vi "newUser.vi"() -> ()   [LabVIEW 2020, in "userLibrary.lvlib"]
uses:
  userLibrary.lvlib
  <vilib>/measure/mamon.llb/Trigger Detection for 1 Channel.vi
  <vilib>/addons/database/Connection.llb/DB Tools Open Connec (String).vi
  <vilib>/addons/database/_DB Variant To Data/Database Variant To Data.xnode
  <vilib>/addons/database/NI_Database_API.lvlib
  databaseLibrary.lvlib
  maintenanceLibrary.lvlib
  <vilib>/measure/NI_MAPro.lvlib
panel:
  out "status 2":bool
  out "status 1":bool
  out "Log Max row":i32
  in  "Cancel":bool
  in  "OK":bool
  in  "Is Admin?":enum32{"Yes", "No"}(radio)
  in  "Full Name":string
  in  "Confirm Password":string
  in  "Password":string
  in  "Username":string
  # "New User"
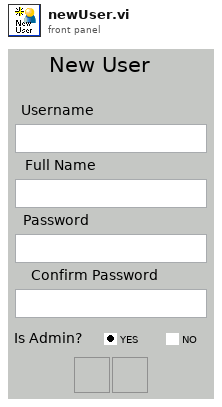
[diagram p1: front panel]
types:
  T1 = typedef "NI_Database_API.lvlib/Conn ObjectReference.ctl" = refnum<k1>
  T2 = cluster{"concatenated string":string, "date/time string":string, "date/time string":string, string}
  T3 = cluster{"Username":string, "Full Name":string, "Password":string, string}
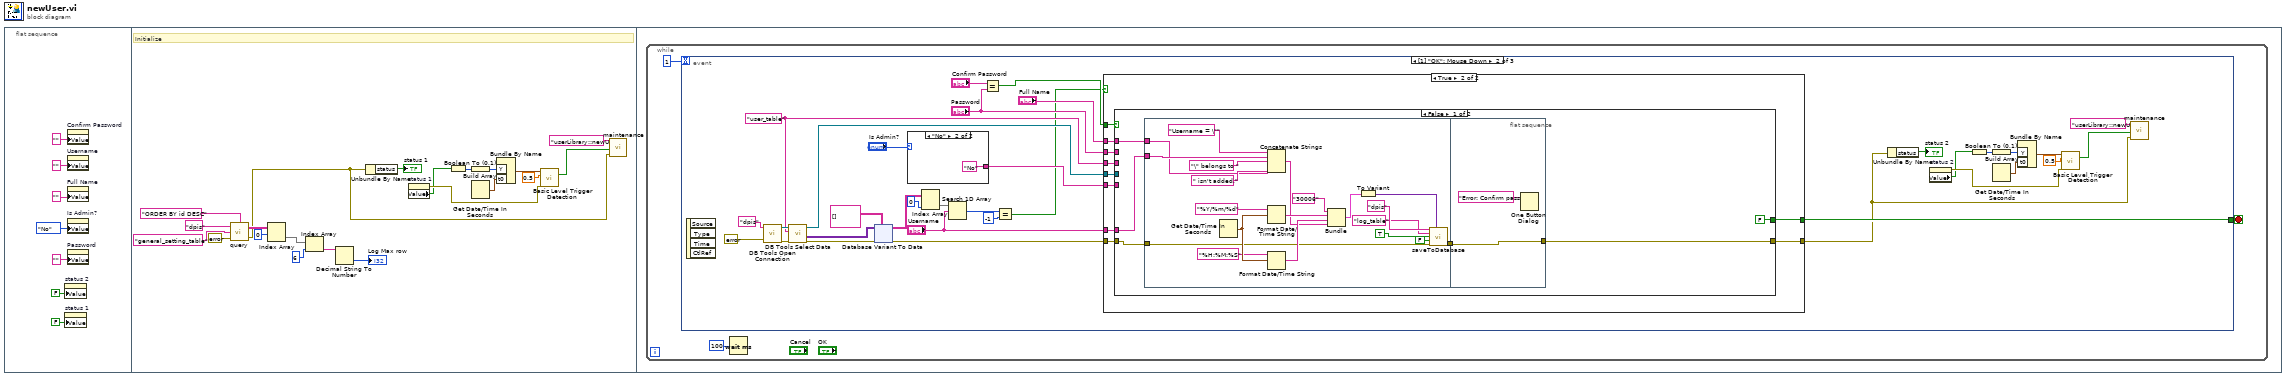
[diagram p0: block diagram]
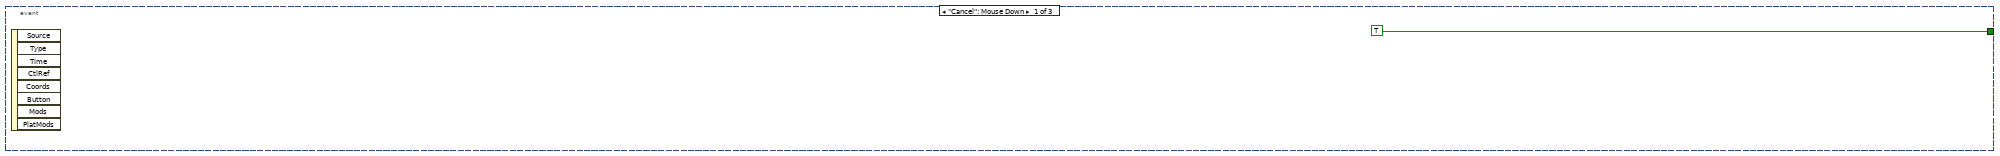
[diagram p2: hidden frame]
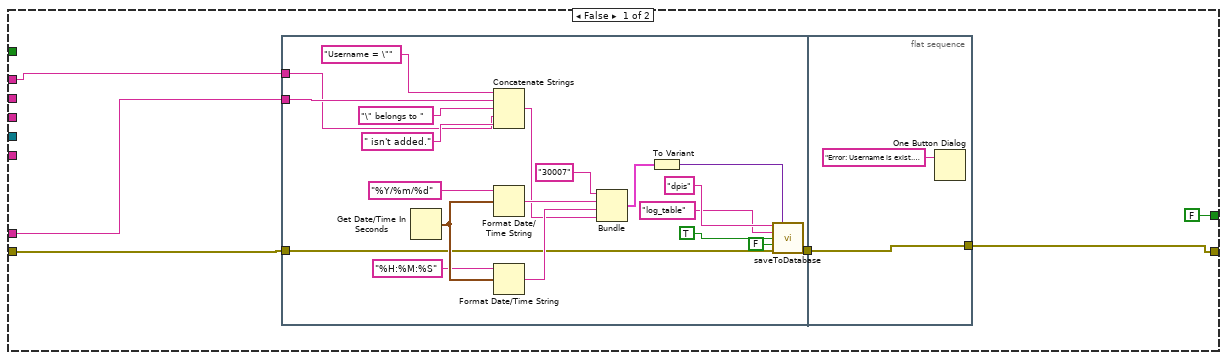
[diagram p3: hidden frame]
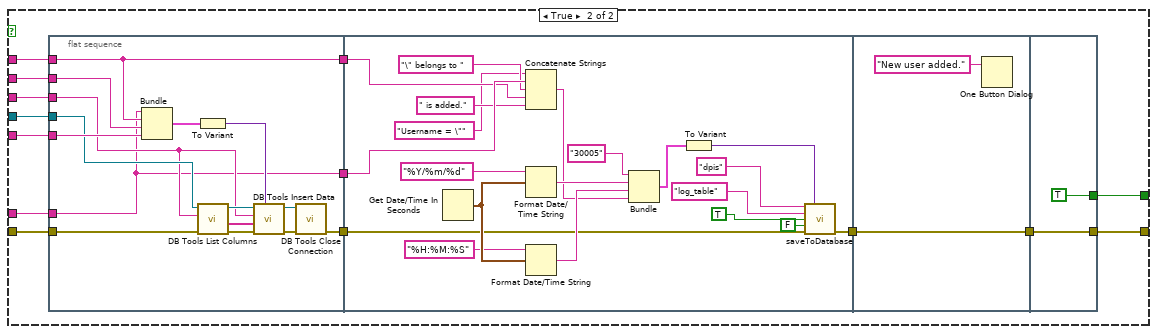
[diagram p4: hidden frame]
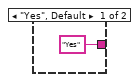
[diagram p5: hidden frame]
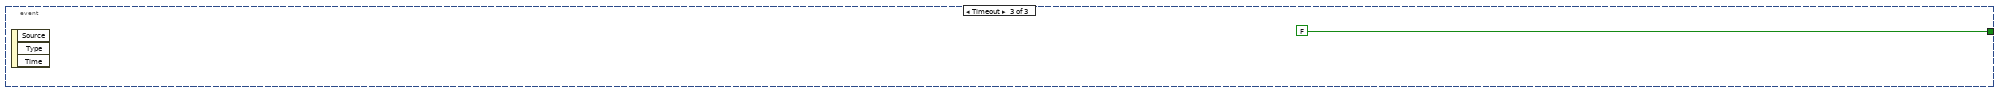
[diagram p6: hidden frame]
diagram:
  n1 = flat-sequence {
    frame #0 {
      n2 = property on="status 2" class="Bool (strict)"("Value"=FALSE ("status 2")) -> ()  [unwired: 2 in, 2 out]
      n3 = property on="status 1" class="Bool (strict)"("Value"=FALSE ("status 1")) -> ()  [unwired: 2 in, 2 out]
      n4 = property on="Confirm Password" class="Str"("Value"="" ("Username")) -> ()  [unwired: 2 in, 2 out]
      n5 = property on="Username" class="Str"("Value"="" ("Username")) -> ()  [unwired: 2 in, 2 out]
      n6 = property on="Full Name" class="Str"("Value"="" ("Full Name")) -> ()  [unwired: 2 in, 2 out]
      n7 = property on="Is Admin?" class="RadioBtnsControl (strict)"("Value"=enum32{"Yes", "No"}."No" ("Is Admin?")) -> ()  [unwired: 2 in, 2 out]
      n8 = property on="Password" class="Str"("Value"="" ("Username")) -> ()  [unwired: 2 in, 2 out]
    }
    frame #1 {
      # "Initialize"
      n9 = call "query.vi"("Condition"="ORDER BY id DESC", "errorIn"=errorcluster {"status"=FALSE, "code"=0, "source"=""} ("Error in"), "Table Name"="general_setting_table", "Connection Name"="dpis") -> ("errorOut"=w8:errorcluster, "data"=w28:string[][])
      n10 = Index Array(array=w28, index (row)=0) -> (element=w27:string[])  [unwired: 1 in]
      n11 = Index Array(array=w27, index=6) -> (element=w26:string)
      n12 = Decimal String To Number(string=w26) -> (number=→"Log Max row":i32)  [unwired: 2 in, 1 out]
      n13 = Unbundle By Name(w8) -> ("status"=→"status 1":bool)
      n14 = property on="status 1" class="Bool (strict)"() -> (error out=w16:errorcluster, "Value"=w15:bool)  [unwired: 2 in, 1 out]
      n15 = Boolean To (0,1)(Boolean=w15) -> (0, 1=w11:i16)
      n16 = Build Array(w11) -> (w13:i16[])
      n17 = Get Date/Time In Seconds() -> (seconds since 1Jan1904=w12:timestamp)
      n18 = Bundle By Name("Y"=w13, "t0"=w12) -> (w14:waveform(i16))  [unwired: 1 in]
      n19 = call-poly <vilib>:"Basic Level Trigger Detection.vi"("signal in"=w14, "level"=0.5, "error in (no error)"=w16) -> ("trigger detected?"=w17:bool)  [unwired: 10 in, 2 out]
      n20 = call "maintenance.vi"("errorIn"=w8, "status"=w17, "errorLocation"="userLibrary::newUser.vi::Initialize") -> ()  [unwired: 8 in, 1 out]
    }
    frame #2 {
      n21 = while {
        stop <- w30 stop-if-true
        n22 = event shown="[1] \"OK\": Mouse Down" {
          selector: _ -> [_ _ _]
          dyn-events: _ -> [_ _ _]
          timeout: 1 -> [_ _ _]
          tunnel: [TRUE w44 FALSE] -> w30
          event "Cancel": Mouse Down {
            n23 = event-data() -> ()  [unwired: 1 in, 8 out]
          }
          event "OK": Mouse Down {
            w57 = "user_table" ("Heat Table Name")
            n24 = event-data() -> ()  [unwired: 1 in, 4 out]
            n25 = call-poly <vilib>:"DB Tools Open Connection.vi"("error in (no error)"=errorcluster {"status"=FALSE, "code"=0, "source"=""}, "connection information"="dpis" ("Connection Name")) -> ("error out"=w61:errorcluster, "connection reference"=w60:T1)  [unwired: 6 in]
            n26 = call <vilib>:"DB Tools Select Data.vi"("error in (no error)"=w61, "table"=w57, "connection reference"=w60) -> ("error out"=w55:errorcluster, "data"=w56:variant[][], "connection reference out"=w58:T1)  [unwired: 3 in]
            n27 = xnode "Database Variant To Data"("database variant"=w56, "error in (no error)"=w55, "type"=string[][] []) -> ("data"=w52:string[][], "error out"=w54:errorcluster)
            n28 = case shown="\"No\"" "Is Admin?" {
              tunnel: ["Yes" "No"] -> w62
              frame "Yes", Default {
              }
              frame "No" {
              }
            }
            n29 = Index Array(array=w52, index (col)=0 ("disabled index (col)")) -> (element=w50:string[])  [unwired: 1 in]
            n30 = Search 1D Array(1D array=w50, element="Username") -> (index of element=w48:i32)  [unwired: 1 in]
            n31 = Equal?(x="Confirm Password", y="Password") -> (x = y?=w65:bool)
            n32 = Equal?(x=w48, y=-1) -> (x = y?=w46:bool)
            n33 = case shown="True" w46 {
              tunnel: w65 -> [_ w105]
              tunnel: "Full Name" -> [w69 w104]
              tunnel: "Password" -> [_ w103]
              tunnel: w62 -> [_ w102]
              tunnel: [FALSE w101] -> w44
              tunnel: w58 -> [_ w100]
              tunnel: [w70 w96] -> w33
              tunnel: w57 -> [_ w99]
              tunnel: w54 -> [w71 w98]
              tunnel: "Username" -> [w68 w97]
              frame False {
                n34 = flat-sequence {
                  tunnel: w68 -> [w78]
                  tunnel: w69 -> [w77]
                  tunnel: w71 -> [w76]
                  tunnel: [w75] -> w72
                  tunnel: [w95] -> w70
                  tunnel: w72 -> [w95]
                  frame #0 {
                    n35 = Get Date/Time In Seconds() -> (seconds since 1Jan1904=w89:timestamp)
                    n36 = Concatenate Strings("Username = \"" ("string"), w78, "\" belongs to " ("string"), w77, " isn't added." ("string")) -> (w88:string)
                    n37 = Format Date/Time String(time format string (%c)="%Y/%m/%d", seconds (now)=w89) -> (date/time string=w90:string)  [unwired: 1 in]
                    n38 = Format Date/Time String(time format string (%c)="%H:%M:%S", seconds (now)=w89) -> (date/time string=w91:string)  [unwired: 1 in]
                    n39 = Bundle("concatenated string"="30007", "date/time string"=w90, "date/time string"=w91, w88) -> (w92:T2)  [unwired: 1 in]
                    n40 = To Variant(anything=w92) -> (Variant=w93:variant)
                    n41 = call "saveToDatabase.vi"("Connection"="dpis" ("table"), "Data"=w93, "Table"="log_table" ("table"), "Auto Increment ID?"=TRUE, "Delete row?"=FALSE, "Error in"=w76) -> ("Error out"=w75:errorcluster)  [unwired: 9 in]
                  }
                  frame #1 {
                    n42 = One Button Dialog(message="Error: Username is exist. Please choose another username.") -> ()  [unwired: 1 in, 1 out]
                  }
                }
              }
              frame True {
                n43 = case shown="False" w105 {
                  tunnel: w97 -> [w110 w147]
                  tunnel: w104 -> [w109 w146]
                  tunnel: w103 -> [_ w145]
                  tunnel: w102 -> [_ w144]
                  tunnel: [FALSE w140] -> w101
                  tunnel: w98 -> [w108 w143]
                  tunnel: w100 -> [_ w142]
                  tunnel: [w107 w136] -> w96
                  tunnel: w99 -> [_ w141]
                  frame False {
                    n44 = flat-sequence {
                      tunnel: w110 -> [w116]
                      tunnel: w109 -> [w115]
                      tunnel: w108 -> [w114]
                      tunnel: [w113] -> w106
                      tunnel: [w132] -> w107
                      tunnel: w106 -> [w132]
                      frame #0 {
                        n45 = Get Date/Time In Seconds() -> (seconds since 1Jan1904=w127:timestamp)
                        n46 = Concatenate Strings("Username = \"" ("string"), w116, "\" belongs to " ("string"), w115, " isn't added." ("string")) -> (w126:string)
                        n47 = Format Date/Time String(time format string (%c)="%Y/%m/%d", seconds (now)=w127) -> (date/time string=w128:string)  [unwired: 1 in]
                        n48 = Format Date/Time String(time format string (%c)="%H:%M:%S", seconds (now)=w127) -> (date/time string=w129:string)  [unwired: 1 in]
                        n49 = Bundle("concatenated string"="30006", "date/time string"=w128, "date/time string"=w129, w126) -> (w130:T2)  [unwired: 1 in]
                        n50 = To Variant(anything=w130) -> (Variant=w131:variant)
                        n51 = call "saveToDatabase.vi"("Connection"="dpis" ("table"), "Data"=w131, "Table"="log_table" ("table"), "Auto Increment ID?"=TRUE, "Delete row?"=FALSE, "Error in"=w114) -> ("Error out"=w113:errorcluster)  [unwired: 9 in]
                      }
                      frame #1 {
                        n52 = One Button Dialog(message="Error: Confirm password does not match.") -> ()  [unwired: 1 in, 1 out]
                      }
                    }
                  }
                  frame True {
                    n53 = flat-sequence {
                      tunnel: w147 -> [w151]
                      tunnel: w146 -> [w152]
                      tunnel: w145 -> [w162]
                      tunnel: w144 -> [w161]
                      tunnel: w143 -> [w156]
                      tunnel: w142 -> [w155]
                      tunnel: w141 -> [w153]
                      tunnel: [w152] -> w139
                      tunnel: [w151] -> w138
                      tunnel: [w149] -> w137
                      tunnel: w139 -> [w171]
                      tunnel: w138 -> [w173]
                      tunnel: w137 -> [w168]
                      tunnel: [w167] -> w134
                      tunnel: [w183] -> w135
                      tunnel: w134 -> [w183]
                      tunnel: [TRUE] -> w140
                      tunnel: [w185] -> w136
                      tunnel: w135 -> [w185]
                      frame #0 {
                        n54 = Bundle("Username"=w151, "Full Name"=w152, "Password"=w162, w161) -> (w157:T3)  [unwired: 1 in]
                        n55 = To Variant(anything=w157) -> (Variant=w160:variant)
                        n56 = call <vilib>:"DB Tools List Columns.vi"("error in (no error)"=w156, "table"=w153, "connection reference"=w155) -> ("error out"=w159:errorcluster, "columns"=w148:string[], "connection reference out"=w158:T1)  [unwired: 1 in, 1 out]
                        n57 = call <vilib>:"DB Tools Insert Data.vi"("data"=w160, "error in (no error)"=w159, "columns"=w148, "table"=w153, "connection reference"=w158) -> ("error out"=w150:errorcluster, "connection reference out"=w154:T1)  [unwired: 5 in]
                        n58 = call <vilib>:"DB Tools Close Connection.vi"("error in (no error)"=w150, "connection reference"=w154) -> ("error out"=w149:errorcluster)  [unwired: 5 in]
                      }
                      frame #1 {
                        n59 = Get Date/Time In Seconds() -> (seconds since 1Jan1904=w178:timestamp)
                        n60 = Concatenate Strings("Username = \"" ("string"), w173, "\" belongs to " ("string"), w171, " is added." ("string")) -> (w169:string)
                        n61 = Format Date/Time String(time format string (%c)="%Y/%m/%d", seconds (now)=w178) -> (date/time string=w179:string)  [unwired: 1 in]
                        n62 = Format Date/Time String(time format string (%c)="%H:%M:%S", seconds (now)=w178) -> (date/time string=w180:string)  [unwired: 1 in]
                        n63 = Bundle("concatenated string"="30005", "date/time string"=w179, "date/time string"=w180, w169) -> (w181:T2)  [unwired: 1 in]
                        n64 = To Variant(anything=w181) -> (Variant=w182:variant)
                        n65 = call "saveToDatabase.vi"("Connection"="dpis" ("table"), "Data"=w182, "Table"="log_table" ("table"), "Auto Increment ID?"=TRUE, "Delete row?"=FALSE, "Error in"=w168) -> ("Error out"=w167:errorcluster)  [unwired: 9 in]
                      }
                      frame #2 {
                        n66 = One Button Dialog(message="New user added.") -> ()  [unwired: 1 in, 1 out]
                      }
                      frame #3 {
                      }
                    }
                  }
                }
              }
            }
            n67 = Unbundle By Name(w33) -> ("status"=→"status 2":bool)
            n68 = property on="status 2" class="Bool (strict)"() -> (error out=w41:errorcluster, "Value"=w40:bool)  [unwired: 2 in, 1 out]
            n69 = Boolean To (0,1)(Boolean=w40) -> (0, 1=w36:i16)
            n70 = Build Array(w36) -> (w38:i16[])
            n71 = Get Date/Time In Seconds() -> (seconds since 1Jan1904=w37:timestamp)
            n72 = Bundle By Name("Y"=w38, "t0"=w37) -> (w39:waveform(i16))  [unwired: 1 in]
            n73 = call-poly <vilib>:"Basic Level Trigger Detection.vi"("signal in"=w39, "level"=0.5, "error in (no error)"=w41) -> ("trigger detected?"=w42:bool)  [unwired: 10 in, 2 out]
            n74 = call "maintenance.vi"("errorIn"=w33, "status"=w42, "errorLocation"="userLibrary::newUser.vi::OK case") -> ()  [unwired: 8 in, 1 out]
          }
          event Timeout {
            n75 = event-data() -> ()  [unwired: 1 in, 3 out]
          }
        }
        n76 = Wait (ms)(milliseconds to wait=u32 100) -> ()  [unwired: 1 out]
      }
    }
  }
